vi "Test Helper Loop Broadcast Started State.vi"(8 "error in (no error)":errorcluster, 11 "Helper Loop Test In":refnum<class "Helper Loop Test.lvclass">) -> (0 "error out":errorcluster, 3 "Helper Loop Test Out":refnum<class "Helper Loop Test.lvclass">)   [LabVIEW 2020, in "Helper Loop Test.lvclass"]
uses:
  Helper Loop Test.lvclass
  C:/Program Files (x86)/National Instruments/LabVIEW 2020/vi.lib/Astemes/LUnit/Test Case.lvclass
  source/Framework Test Suite/Mock Process/Mock Process.lvclass
  C:/git/astemes-triarc-framework/source/Framework/Process/Process.lvclass
  source/Framework/Process/Process.lvclass/Process.ctl
  <vilib>/Astemes/LUnit/Test Case.lvclass/Test Case.ctl
  45129f09-3b7f-4dca-a147-c80fc5177134.vi
  source/Framework/Process/Public/Lifecycle/Get Lifecycle State.vi
  source/Framework/Broadcast Event Helpers/Execution timer.vi
  source/Framework/Process/Private/SubVIs/Wait for finish.vi
  source/Framework/Process/Private/SubVIs/Set Lifecycle State.vi
  source/Framework/Process/Protected/Messaging/Send Message.vi
  <vilib>/Astemes/LUnit/Append Pass Result.vi
  <vilib>/Astemes/LUnit/Append Fail Result.vi
  <vilib>/Astemes/LUnit/Describe Comparison.vi
  <vilib>/Astemes/LUnit/Compare Variants.vi
  <vilib>/Utility/error.llb/Clear Errors.vi
  source/Framework/Process/Private/SubVIs/Handle Debug Data.vi
  <vilib>/Astemes/LUnit/Variant to string.vi
  source/Framework/Logging/Log Debug.vi
  <vilib>/AdvancedString/1D String Array to Delimited String.vi
  <vilib>/Utility/High Resolution Relative Seconds.vi
  <vilib>/Utility/error.llb/Error Cluster From Error Code.vi
  source/Framework/Broadcast Event Dequeuers/Dequeue Broadcast Message.vi
  source/Framework/Process/Public/Read Name.vi
  <vilib>/Utility/Data Type/Get Type Information.vi
  <vilib>/Utility/LVClass/Get LV Class Name.vi
  source/Framework/Callback/Callback.lvclass
  source/Framework/Process/Process.lvclass
  Helper Loop Test.lvclass/Helper Loop Test.ctl
  source/Framework/Broadcast Event Dequeuers/Broadcast Event Dequeuers.lvlib
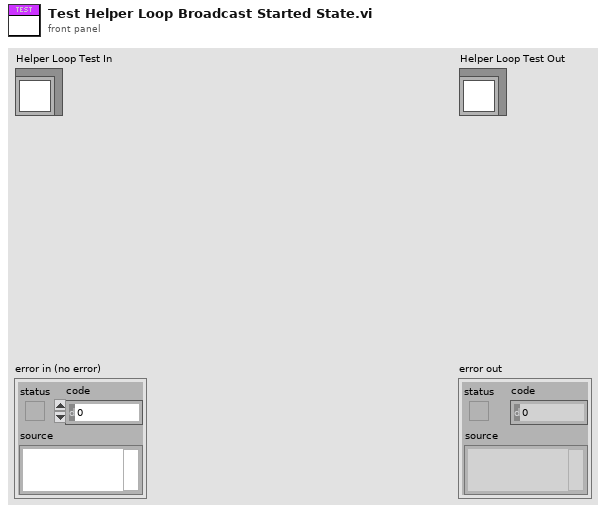
[diagram p1: front panel]
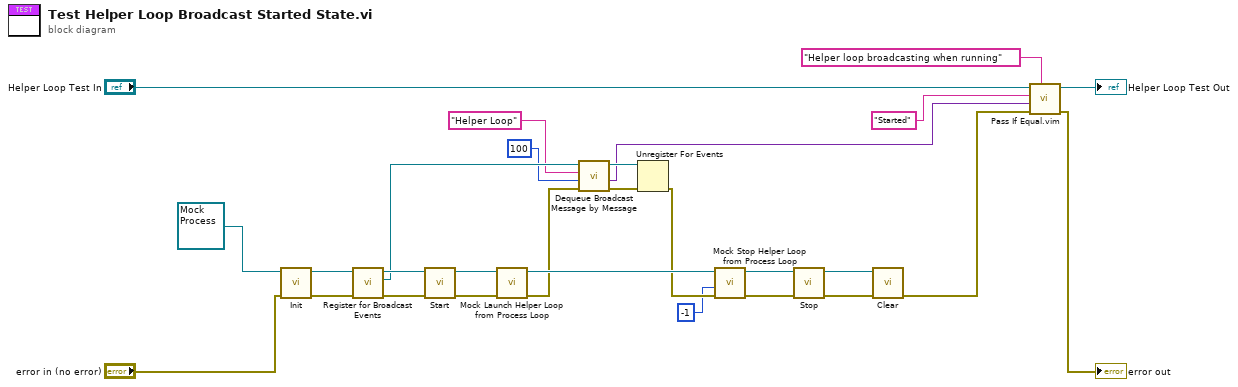
[diagram p0: block diagram]
diagram:
  n1 = call-dynamic "Init.vi"("error in (no error)"="error in (no error)", "Mock Process In"=refnum<class "Mock Process.lvclass"> refnum) -> ("error out"=w26:errorcluster, "Mock Process Out"=w27:refnum<class "Mock Process.lvclass">)  [unwired: 8 in]
  n2 = call "Register for Broadcast Events.vi"("error in (no error)"=w26, "Process In"=w27) -> ("error out"=w24:errorcluster, "Event Registration Refnum Out"=w11:refnum<event-registration>, "Process Out"=w25:refnum<class "Mock Process.lvclass">)  [unwired: 7 in]
  n3 = call "Start.vi"("error in (no error)"=w24, "Process In"=w25) -> ("error out"=w22:errorcluster, "Process Out"=w23:refnum<class "Mock Process.lvclass">)  [unwired: 7 in, 1 out]
  n4 = call "Mock Launch Helper Loop from Process Loop.vi"("error in (no error)"=w22, "Mock Process in"=w23) -> ("error out"=w9:errorcluster, "Mock Process out"=w21:refnum<class "Mock Process.lvclass">)  [unwired: 8 in]
  n5 = call "Dequeue Broadcast Message by Message.vi"("error in (no error)"=w9, "Timeout (-1)"=100, "Message"="Helper Loop" ("y"), "Event Registration Refnum"=w11) -> ("error out"=w3:errorcluster, "Message Data"=w2:variant, "Event Registration Refnum Out"=w8:refnum<event-registration>)  [unwired: 3 in, 2 out]
  n6 = Unregister For Events(event registration refnum=w8, error in=w3) -> (error out=w7:errorcluster)
  n7 = call "Mock Stop Helper Loop from Process Loop.vi"("error in (no error)"=w7, "timeout in ms (-1)"=-1, "Mock Process in"=w21) -> ("error out"=w19:errorcluster, "Mock Process out"=w20:refnum<class "Mock Process.lvclass">)  [unwired: 6 in, 1 out]
  n8 = call "Stop.vi"("error in (no error)"=w19, "Process In"=w20) -> ("error out"=w18:errorcluster, "Process Out"=w1:refnum<class "Mock Process.lvclass">)  [unwired: 7 in, 1 out]
  n9 = call-dynamic "Clear.vi"("error in (no error)"=w18, "Mock Process In"=w1) -> ("error out"=w17:errorcluster)  [unwired: 9 in]
  n10 = call "Pass If Equal.vim"("Description"="Helper loop broadcasting when running", "error in (no error)"=w17, "Actual"=w2, "Expected"="Started" ("Description"), "LUnit Test Case In"="Helper Loop Test In") -> ("error out"=→"error out":errorcluster, "LUnit Test Case Out"=→"Helper Loop Test Out":refnum<class "Helper Loop Test.lvclass">)  [unwired: 5 in]
